vi "acquisitionSaveFrames.vi"(1 "frames (1D)":u16[](array[numeric])) -> ()   [LabVIEW 2017]
uses:
  globalUtilities.vi
  globalDevices.vi
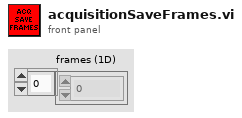
[diagram p1: front panel]
types:
  T1 = enum16{"big-endian, network order", "native, host order", "little-endian"}
  T2 = enum16{"open", "replace", "create", "open or create", "replace or create", "replace or create with confirmation"}
  T3 = cluster{"height":i32, "width":i32, "datatype":i32}
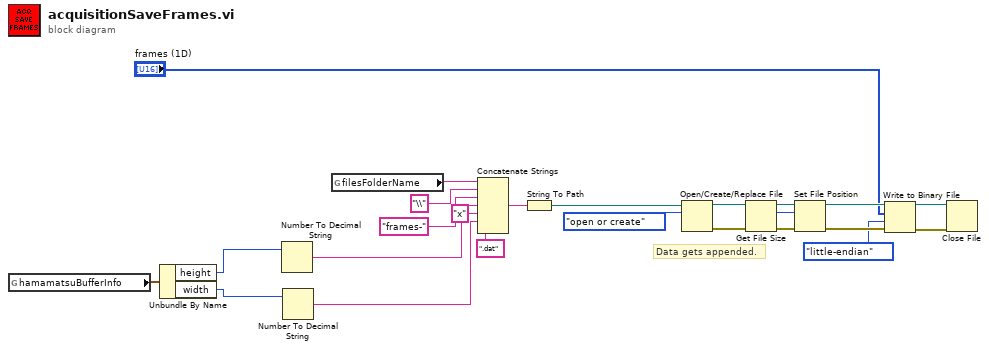
[diagram p0: block diagram]
diagram:
  # "Data gets appended."
  n1 = global read "globalDevices.vi" "hamamatsuBufferInfo"() -> (w4:T3)
  n2 = Unbundle By Name(w4) -> ("height"=w3:i32, "width"=w2:i32)
  n3 = Number To Decimal String(number=w3) -> (decimal integer string=w21:string)  [unwired: 1 in]
  n4 = Number To Decimal String(number=w2) -> (decimal integer string=w19:string)  [unwired: 1 in]
  n5 = global read "globalUtilities.vi" "filesFolderName"() -> (w24:string)
  n6 = Concatenate Strings(w24, "\\" ("string"), "frames-" ("string"), w21, "x" ("string"), w19, ".dat" ("string")) -> (w17:string)
  n7 = String To Path(string=w17) -> (path=w16:path)
  n8 = Open/Create/Replace File(file path (use dialog)=w16, operation (0:open)=T2."open or create") -> (refnum out=w14:refnum<file>, error out=w13:errorcluster)  [unwired: 4 in, 1 out]
  n9 = Get File Size(file=w14, error in=w13) -> (refnum out=w12:refnum<file>, size (in bytes)=w10:i64, 0:w11:errorcluster)
  n10 = Set File Position(offset (in bytes) (0)=w10, refnum=w12, error in=w11) -> (refnum out=w9:refnum<file>, error out=w8:errorcluster)  [unwired: 1 in]
  n11 = Write to Binary File(file (use dialog)=w9, data="frames (1D)", error in=w8, 9:T1."little-endian" ("byte order (0:big-endian, network order)")) -> (refnum out=w6:refnum<file>, error out=w5:errorcluster)  [unwired: 2 in, 1 out]
  n12 = Close File(refnum=w6, error in=w5) -> ()  [unwired: 2 out]
